vi "Set CANopen Master Node-ID.vi"(8 "error in":errorcluster, 10 "Node-ID":u8=127 format="0x%02x", 11 "Interactor in":refnum<class "Interactor.lvclass">) -> (0 "error out":errorcluster, 3 "Interactor out":refnum<class "Interactor.lvclass">)   [LabVIEW 2024, in "Interactor.lvlib" / "Interactor.lvclass"]
uses:
  Interactor.lvclass
  Interactor.lvclass/Interactor.ctl
  CANopen Master/CANopen Master.lvclass
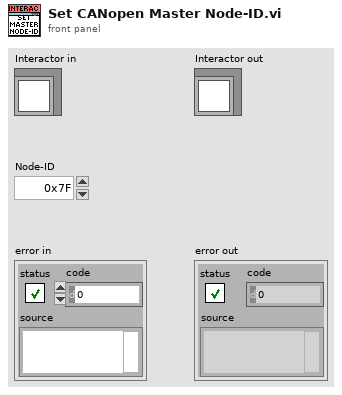
[diagram p1: front panel]
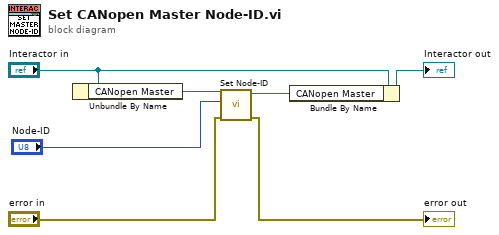
[diagram p0: block diagram]
diagram:
  n1 = Unbundle By Name("Interactor in") -> ("CANopen Master"=w6:refnum<class "CANopen Master.lvclass">)
  n2 = call "Set Node-ID.vi"("error in"="error in", "Node-ID"="Node-ID", "CANopen Master in"=w6) -> ("error out"=→"error out":errorcluster, "CANopen Master out"=w1:refnum<class "CANopen Master.lvclass">)  [unwired: 7 in]
  n3 = Bundle By Name(cluster="Interactor in", "CANopen Master"=w1) -> (→"Interactor out":refnum<class "Interactor.lvclass">)
